vi "GetAttrib.vi"(0 "Device in":refnum<class "Device.lvclass">, 11 "error in (no error)":errorcluster) -> (1 "Mec NegLim":string, 2 "Mec PosLim":string, 3 "Mec Speed":dbl, 4 "Device out":refnum<class "Device.lvclass">, 5 "Mec ID":string, 6 "MecTargets":dbl[](array[numeric])=[0.0, 4.0, 34.0, 64.5, 95.0, 125.5], 7 "MecOffset":string, 8 "MecTarget":dbl caption="Target" min=-1.0 max=131.0 step=0.001 format="%.2f", 10 "VISA Mec":refnum<visa-resource-name>="COM6", 12 "MecEnabled":bool=TRUE, 13 "Mec Factor":dbl, 14 "Mec Acceleration":dbl, 15 "error out":errorcluster)   [LabVIEW 2012]
uses:
  Device.lvclass
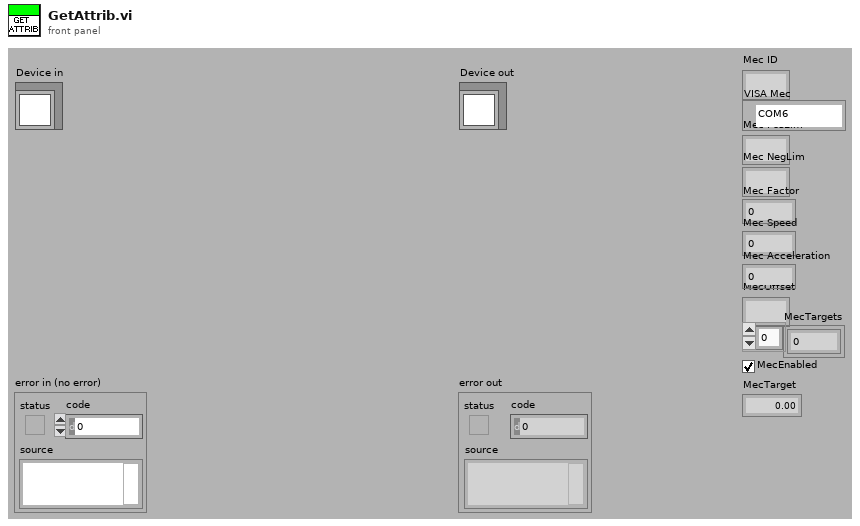
[diagram p1: front panel]
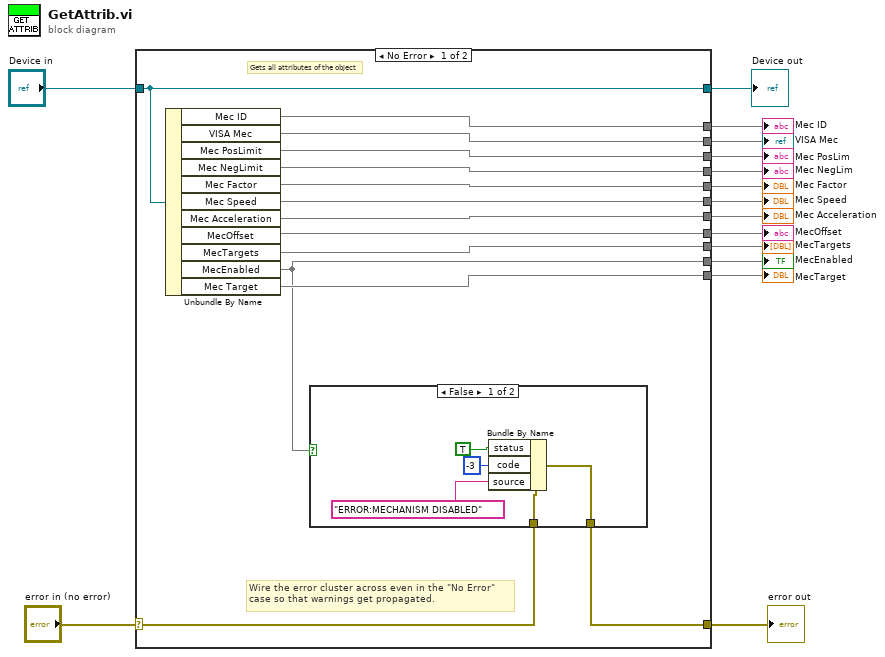
[diagram p0: block diagram]
diagram:
  n1 = case shown="No Error" "error in (no error)" {
    selector: "error in (no error)" -> [w18 w37]
    tunnel: [w17 w37] -> w14
    tunnel: [w29 w36] -> w12
    tunnel: "Device in" -> [w29 w36]
    tunnel: [w28 _] -> w11
    tunnel: [w27 _] -> w10
    tunnel: [w26 _] -> w9
    tunnel: [w25 _] -> w8
    tunnel: [w24 _] -> w7
    tunnel: [w23 _] -> w6
    tunnel: [w22 _] -> w5
    tunnel: [w21 _] -> w4
    tunnel: [w20 _] -> w3
    tunnel: [w16 _] -> w2
    tunnel: [w19 _] -> w1
    frame No Error {
      # "Gets all attributes of the object"
      # "Wire the error cluster across even in the \"No Error\"\ncase so that warnings get propagated."
      n2 = Unbundle By Name(w29) -> ("Mec ID"=w28, "VISA Mec"=w27, "Mec PosLimit"=w26, "Mec NegLimit"=w25, "Mec Factor"=w24, "Mec Speed"=w23, "Mec Acceleration"=w22, "MecOffset"=w21, "MecTargets"=w20, "MecEnabled"=w16, "Mec Target"=w19)
      n3 = case shown="False" w16 {
        tunnel: w18 -> [w34 w35]
        tunnel: [w33 w35] -> w17
        frame False {
          n4 = Bundle By Name(cluster=w34, "status"=TRUE, "code"=-3, "source"="ERROR:MECHANISM DISABLED") -> (w33:errorcluster)
        }
        frame True {
        }
      }
    }
    frame Error {
      # "Error detected earlier: bypass"
    }
  }
  "error out" <- w14
  "Device out" <- w12
  "Mec ID" <- w11
  "Mec PosLim" <- w9
  "Mec NegLim" <- w8
  "MecOffset" <- w4
  "Mec Factor" <- w7
  "Mec Speed" <- w6
  "Mec Acceleration" <- w5
  "VISA Mec" <- w10
  "MecTargets" <- w3
  "MecEnabled" <- w2
  "MecTarget" <- w1
